vi "BodeMagnitudePlot.vi"() -> ()   [LabVIEW 2014]
uses:
  <vilib>/Analysis/NI_AALPro.lvlib
panel:
  out "XY Graph":cluster{dbl[], i32[]}(graph)
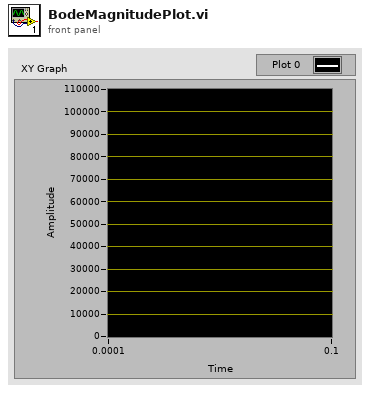
[diagram p1: front panel]
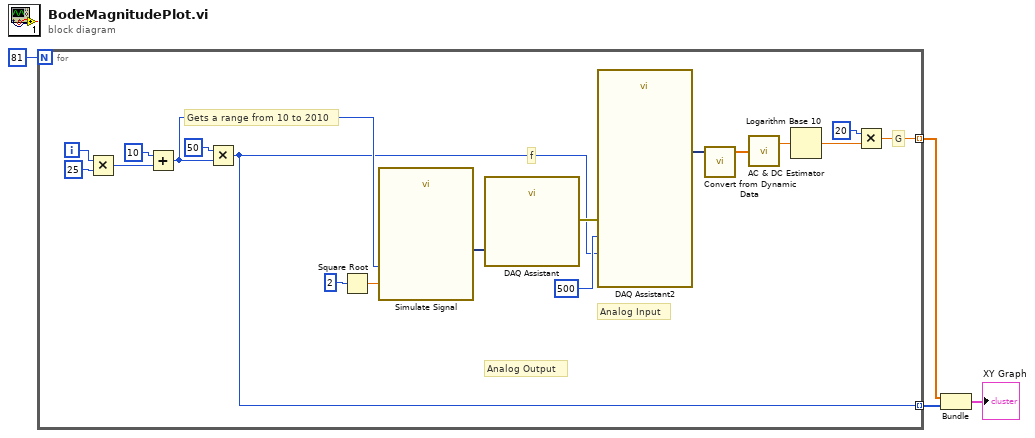
[diagram p0: block diagram]
diagram:
  n1 = for {
    N: 81 -> [_]
    tunnel: [w6] -> w3 mode=indexing
    tunnel: [w5] -> w2 mode=indexing
    i -> [w20]
    # "f"
    # "G"
    # "Analog Input"
    # "Analog Output"
    # "Gets a range from 10 to 2010"
    n2 = Multiply(x=w20, y=25) -> (x*y=w17:i32)
    n3 = Add(x=10, y=w17) -> (x+y=w14:i32)
    n4 = Multiply(x=50, y=w14) -> (x*y=w5:i32)
    n5 = Square Root(x=2) -> (sqrt(x)=w21:dbl)
    n6 = call "Simulate Signal"("Frequency"=w14, "Amplitude"=w21) -> ("Sine"=w16:dynamicdata)  [unwired: 12 in, 1 out]
    n7 = call "DAQ Assistant"("data"=w16) -> ("error out"=w15:errorcluster)  [unwired: 16 in, 2 out]
    n8 = call "DAQ Assistant2"("rate"=w5, "number of samples"=500, "error in"=w15) -> ("data"=w11:dynamicdata)  [unwired: 14 in, 2 out]
    n9 = call "Convert from Dynamic Data"("Dynamic Data Type"=w11) -> ("Array"=w10:dbl[])  [unwired: 3 in]
    n10 = call <vilib>:"AC & DC Estimator.vi"("Signal (V)"=w10) -> ("AC estimate (Vrms)"=w9:dbl)  [unwired: 1 out]
    n11 = Logarithm Base 10(1:w9) -> (0:w7:dbl)
    n12 = Multiply(x=20, y=w7) -> (x*y=w6:dbl)
  }
  n13 = Bundle(w3, w2) -> (→"XY Graph":cluster{dbl[], i32[]})  [unwired: 1 in]
